vi "DWF MSO Query Digital Pattern Trigger.vi"(0 "Instrument Handle In":dbl, 11 "Error In":errorcluster caption="Error In (no error)", 12 "Trigger Instance":i32(ring) caption="Trigger Instance (A)" items=["A", "B"]) -> (4 "Instrument Handle Out":dbl, 6 "Trigger Source":tag, 8 "Trigger Pattern":string, 15 "Error Out":errorcluster)   [LabVIEW 2015, in "DigilentWF.lvlib"]
doc: "Indicates the digital pattern trigger configuration of the specified instance. A trigger is produced when every level (high/low) requirement specified in <B>Trigger Pattern</B> is met, and when at least one toggling (toggle/fall/rise) requirement is met. If no toggling requirements are set, then only the level requirements must be met to produce a trigger."
uses:
  <vilib>/DigilentWF/DigilentWF.lvlib
  dwf.dll
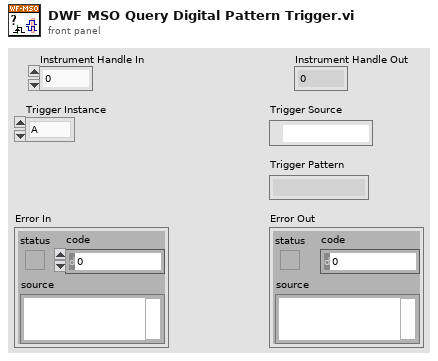
[diagram p1: front panel]
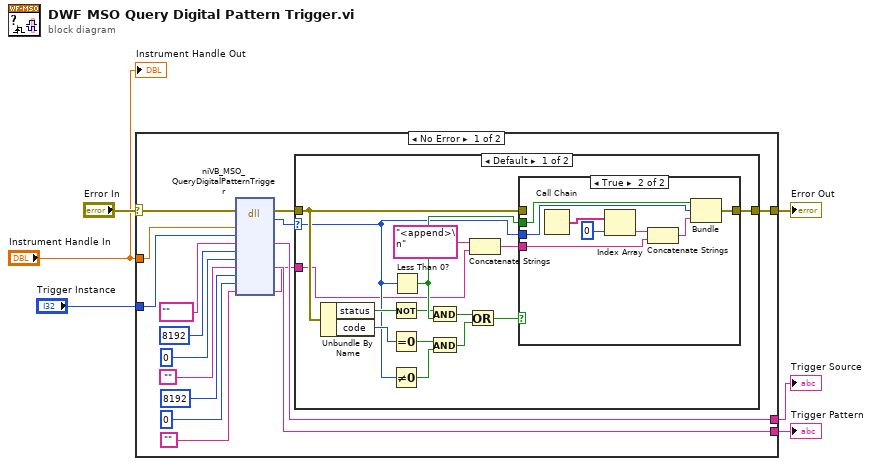
[diagram p0: block diagram]
diagram:
  n1 = case "outter_case" shown="No Error" "Error In" {
    selector: "Error In" -> [w22 w48]
    tunnel: [w19 w48] -> w5
    tunnel: "Instrument Handle In" -> [w18 _]
    tunnel: "Trigger Instance" -> [w17 _]
    tunnel: [w14 _] -> w2
    tunnel: [w13 _] -> w1
    frame No Error {
      n2 = dll-call lib="dwf.*" fn="niVB_MSO_QueryDigitalPatternTrigger"(error in=w22, "InstrumentHandle"=w18, "TriggerInstance"=w17, "TriggerSource"=tag "" ("Trigger Source"), "cTriggerSource"=8192, "pTriggerSource"=0, "TriggerPattern"="", "cTriggerPattern"=8192, "pTriggerPattern"=0, "szError"="") -> (error out=w21:errorcluster, "return type"=w20:i32, "TriggerSource"=w14:string, "TriggerPattern"=w13:string, "szError"=w11:string)  [unwired: 8 in, 1 out]
      n3 = case "inner_case" shown="Default" w20 {
        selector: w20 -> [w27 _]
        tunnel: w21 -> [w28 w47]
        tunnel: [w24 w47] -> w19
        tunnel: w11 -> [w23 _]
        frame Default {
          n4 = Unbundle By Name(w28) -> ("status"=w32:bool, "code"=w36:i32)
          n5 = Not(x=w32) -> (.not. x?=w35:bool)
          n6 = Equal To 0?(x=w36) -> (x = 0?=w31:bool)
          n7 = Not Equal To 0?(x=w27) -> (x != 0?=w34:bool)
          n8 = Less Than 0?(x=w27) -> (x < 0?=w37:bool)
          n9 = And(x=w35, y=w37) -> (x .and. y?=w33:bool)
          n10 = And(x=w31, y=w34) -> (x .and. y?=w30:bool)
          n11 = Or(x=w33, y=w30) -> (x .or. y?=w29:bool)
          n12 = Concatenate Strings("<append>\n" ("string"), w23) -> (w26:string)
          n13 = case shown="True" w29 {
            tunnel: [w38 w45] -> w24
            tunnel: w27 -> [_ w44]
            tunnel: w37 -> [_ w43]
            tunnel: w28 -> [w38 _]
            tunnel: w26 -> [_ w39]
            frame False {
            }
            frame True {
              n14 = Call Chain() -> (call chain=w42:string[])
              n15 = Index Array(array=w42, index=0) -> (element=w41:string)
              n16 = Concatenate Strings(w41, w39) -> (w46:string)
              n17 = Bundle(w43, "return type"=w44, w46) -> (w45:cluster{bool, "return type":i32, string})  [unwired: 1 out]
            }
          }
        }
        frame 0 {
        }
      }
    }
    frame Error {
    }
  }
  "Error Out" <- w5
  "Trigger Source" <- w2
  "Trigger Pattern" <- w1
  "Instrument Handle Out" <- "Instrument Handle In"
